vi "SMS Analysis Write Remote Info File.vi"() -> ()   [LabVIEW 2020]
uses:
  SMS Analysis Interface Type Defs/SMS Analysis Remote Info.ctl
  SMS Analysis Interface Type Defs/SMS Analysis Interface Connection Info.ctl
panel:
  in  "Done":bool
  in  "Save File":bool
  in  "Remote Settings":T1
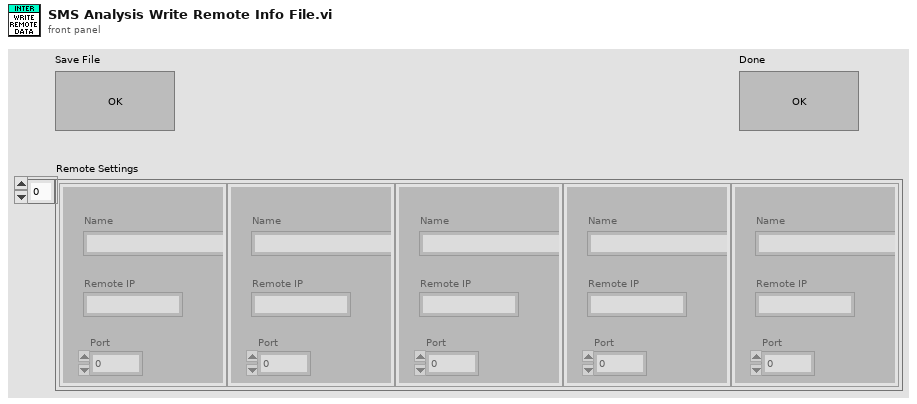
[diagram p1: front panel]
types:
  T1 = typedef "SMS Analysis Remote Info.ctl" = T2[]
  T2 = typedef "SMS Analysis Interface Connection Info.ctl" = cluster{"Name":string, "Remote IP":string, "Port":u16}
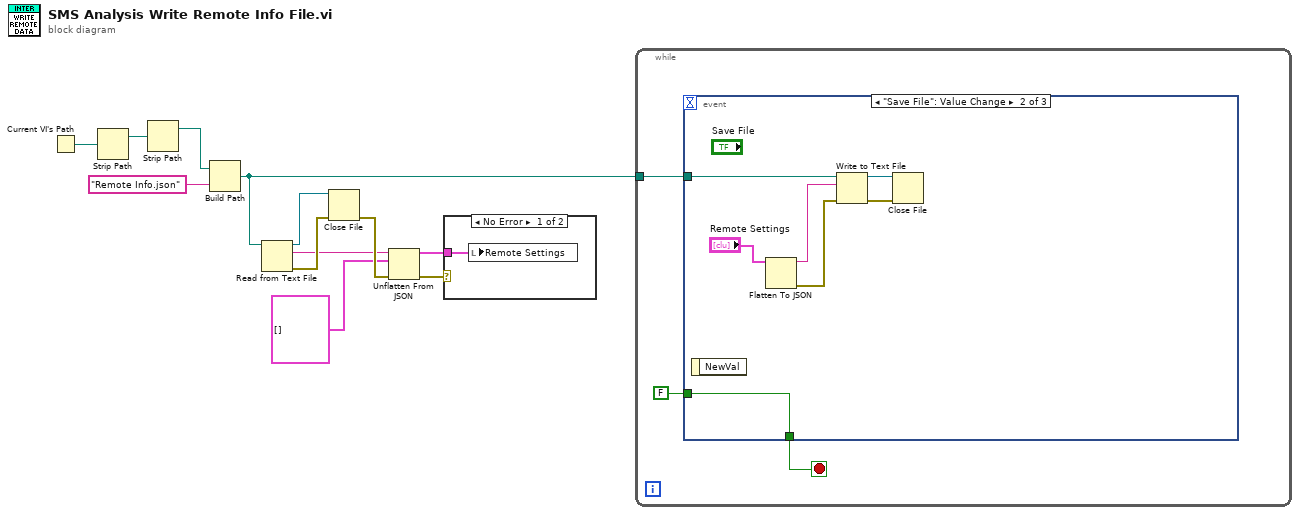
[diagram p0: block diagram]
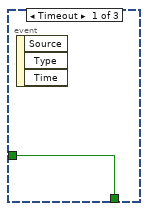
[diagram p3: hidden frame]
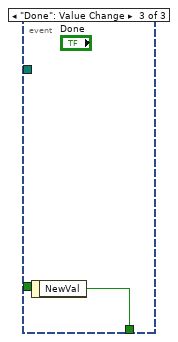
[diagram p4: hidden frame]
diagram:
  n1 = Current VI's Path() -> (path=w12:path)
  n2 = Strip Path(path=w12) -> (stripped path=w11:path)  [unwired: 1 out]
  n3 = Strip Path(path=w11) -> (stripped path=w10:path)  [unwired: 1 out]
  n4 = Build Path(base path=w10, name or relative path="Remote Info.json") -> (appended path=w2:path)
  n5 = Read from Text File(file (use dialog)=w2) -> (refnum out=w8:refnum<file>, text=w5:string, error out=w7:errorcluster)  [unwired: 3 in, 1 out]
  n6 = Close File(refnum=w8, error in=w7) -> (error out=w6:errorcluster)  [unwired: 1 out]
  n7 = Unflatten From JSON(JSON string=w5, type and defaults=T1 [] ("Remote Info"), error in (no error)=w6) -> (value=w3:T1, error out=w4:errorcluster)  [unwired: 4 in]
  n8 = case shown="No Error" w4 {
    tunnel: w3 -> [w13 _]
    frame No Error {
      n9 = local write "Remote Settings"(w13) -> ()
    }
    frame Error {
    }
  }
  n10 = while {
    tunnel: w2 -> [w14]
    stop <- w16 stop-if-true
    n11 = event shown="[1] \"Save File\": Value Change" {
      selector: _ -> [_ _ _]
      dyn-events: _ -> [_ _ _]
      timeout: _ -> [_ _ _]
      tunnel: [w17 w24 w25] -> w16
      tunnel: FALSE -> [w17 w24 _]
      tunnel: w14 -> [_ w22 _]
      event Timeout {
        n12 = event-data() -> ()  [unwired: 1 in, 3 out]
      }
      event "Save File": Value Change {
        n13 = event-data() -> ()  [unwired: 1 in, 1 out]
        n14 = Flatten To JSON(anything="Remote Settings") -> (JSON string=w21:string, 11:w20:errorcluster)  [unwired: 2 in]
        n15 = Write to Text File(file (use dialog)=w22, text=w21, error in=w20) -> (refnum out=w19:refnum<file>, error out=w18:errorcluster)  [unwired: 1 in, 1 out]
        n16 = Close File(refnum=w19, error in=w18) -> ()  [unwired: 2 out]
      }
      event "Done": Value Change {
        n17 = event-data() -> ("NewVal"=w25:bool)  [unwired: 1 in]
      }
    }
  }
